vi "configureILC.vi"(8 "error in (no error)":errorcluster, 10 "ILCConfig":T1 {"ADC PGA Gain" max=7}, 11 "Model in":refnum<class "Model.lvclass">) -> (0 "error out":errorcluster, 3 "Model out":refnum<class "Model.lvclass">)   [LabVIEW 2012, in "Model.lvclass"]
uses:
  Model.lvclass
  Program Files (x86)/National Instruments/LabVIEW 2012/user.lib/Common/ILC/Configuration/ILCConfig.ctl
  Program Files (x86)/National Instruments/LabVIEW 2012/user.lib/Common/ILC/Configuration/InputChannels.ctl
  Program Files (x86)/National Instruments/LabVIEW 2012/user.lib/Common/ILC/Configuration/ScanRate_Hz_MultichannelOptions.ctl
  Model.lvclass/Model.ctl
  Program Files (x86)/National Instruments/LabVIEW 2012/user.lib/Common/SerialProtocols/SerialCommunicator/SerialCommunicator/SerialCommunicator.lvclass
  Program Files (x86)/National Instruments/LabVIEW 2012/user.lib/Common/ILC/ILC/ILC.lvclass
  Program Files (x86)/National Instruments/LabVIEW 2012/user.lib/Common/ILC/Configuration/ILCConfiguration.lvlib
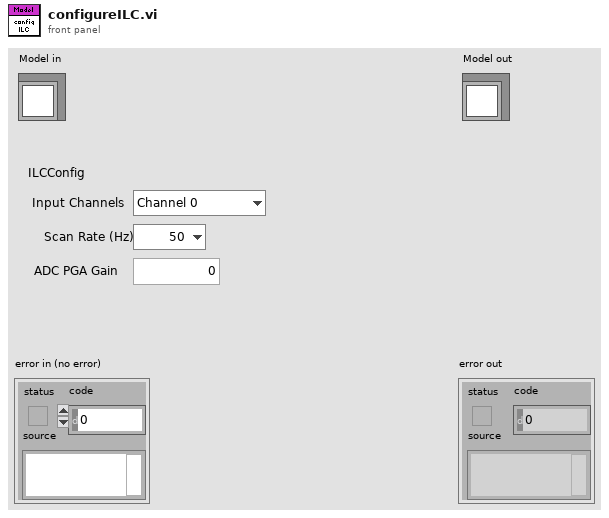
[diagram p1: front panel]
types:
  T1 = typedef "ILCCommon.lvlib/ILCConfiguration.lvlib/ILCConfig.ctl" = cluster{"Input Channels":T2, "Scan Rate (Hz) ":T3, "ADC PGA Gain":u8}
  T2 = typedef "ILCCommon.lvlib/ILCConfiguration.lvlib/InputChannels.ctl" = enum16{"Channel 0", "3 Channels", "5 Channels"}
  T3 = typedef "ILCCommon.lvlib/ILCConfiguration.lvlib/ScanRate_Hz_MultichannelOptions.ctl" = enum16{"50", "60", "100", "120", "200", "240", "300", "400", "480", "600", "1200", "2400", "4800"}
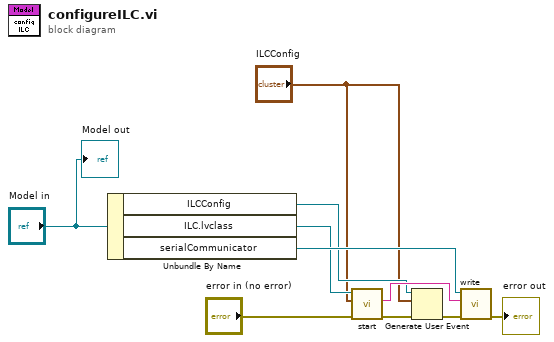
[diagram p0: block diagram]
diagram:
  n1 = Unbundle By Name("Model in") -> ("ILCConfig"=w5:refnum<user-event>, "ILC.lvclass"=w7:refnum<class "ILC.lvclass">, "serialCommunicator"=w9:refnum<class "SerialCommunicator.lvclass">)
  n2 = call "start.vi"("error in (no error)"="error in (no error)", "ILCConfig"="ILCConfig", "ILC in"=w7) -> ("error out"=w2:errorcluster, "configString"=w8:string)  [unwired: 6 in, 1 out]
  n3 = Generate User Event(user event=w5, event data cluster="ILCConfig", error in=w2) -> (error out=w1:errorcluster)  [unwired: 1 out]
  n4 = call-dynamic "write.vi"("error in (no error)"=w1, "writeString"=w8, "SerialCommunicator in"=w9) -> ("error out"=→"error out":errorcluster)  [unwired: 7 in, 1 out]
  "Model out" <- "Model in"
